vi "Gui_SetupExcitation_New.vi"(7 "Variant For Path":variant, 8 "error in (no error)":errorcluster, 11 "Variant":variant) -> (0 "error out":errorcluster caption="sortie d'erreur", 3 "Variant Output":variant)   [LabVIEW 2017]
uses:
  controls/SEQUENCE_Inputs.ctl
  controls/TRAPPING_Inputs.ctl
  controls/EXCIT_Inputs.ctl
  controls/DATA_Inputs.ctl
  controls/TIMING_Inputs.ctl
  controls/PROCESSING_Inputs.ctl
  controls/EXCIT_Form_Selector.ctl
  controls/EXPERT_Inputs.ctl
  controls/DIGIT_5122_Inputs.ctl
  <instrlib>/niScope/Controls/niScope trigger source.ctl
  controls/HSDIO_6541_Inputs.ctl
  <instrlib>/niHSDIO/niHSDIO.llb/niHSDIO_ctl Trigger Source Values (Ring).ctl
  controls/SOFTWARE_Inputs.ctl
  controls/AO_6711_Inputs.ctl
  controls/AWG_5421_Inputs.ctl
  <instrlib>/niFgen/niFgen.llb/niFgen_ctl Trigger Source Values (Ring).ctl
  controls/XML_Inputs.ctl
panel:
  in  "Excit Form":T1=enum."Swift"
  in  "CHECK":bool
  in  "TEST Text":string="script  excit1wfm\n    wait until scriptTrigger0\n    generate E1TwoSwift0p5f1000p0to1002p0a100and1003p0to1004p0a100d1200fs10\n    generate E2Chirp3p5f250p0to1000p0a50d800fs10\n    generate E3TwoSwift0p5f250p0to600p0a70and700p0to1000p0a50d1200fs10\n    generate E4Chirp3p5f250p0to1000p0a50d800fs10\n    generate E5Chirp3p5f250p0to1000p0a50d800fs40\nend script\n"
  in  "Waveforms Table":i32(listbox)
  out "Sampling Frequency":dbl=20.0
  out "Number of Ejects":u16=1
  out "Number of Excits":u16=3
  out "Script Text":string
  in  "SEQUENCE Inputs":T2={"TRAPPING Inputs"={"Number of Channels"=4, "Init Values"=[2.0, 5.0, 5.0, 2.0], "Opening Values"=[0.0, 0.0, 0.0, 0.0], "Trapping Values"=[2.0, 5.0, 5.0, 2.0], "Emptying Values"=[-5.0, -5.0, -5.0, -5.0], "Adiabatic ON"=FALSE, "Adiabatic Duration"=0, "Adiabatic Waveforms"=["Adiabatic_None_2_2_2000.bin", "Adiabatic_Ramp_5_0_2000.bin", "Adiabatic_DoubleRamp_5_0_2000.bin", "Adiabatic_RC_2_0_2000.bin"]}, "EXCIT Inputs"={"Number of Excitations"=1, "Script Text"="", "Table of Waveforms"=[]}, "DATA Inputs"={"Record Length"=8192, "Sample Rate"=4.0, "Data Type"=0, "Vertical Range"=0.0, "Acquisition Duration"=100000.0}, "TIMING Inputs"={"Number of Acquisitions "=1, "Number of Accumulations"=1, "Table of Waveforms"=[], "Script Text"=""}, "PROCESSING Inputs"={"Reference Mass"=300.0939, "Cyclotron Freq"=255.727, "Magnetron Freq"=0.001}} {"PROCESSING Inputs"."Magnetron Freq" format="%.5g"; "PROCESSING Inputs"."Cyclotron Freq" format="%.5g"; "PROCESSING Inputs"."Reference Mass" format="%.5g"; "TIMING Inputs"."Number of Accumulations" min=0 max=50 step=1; "TIMING Inputs"."Number of Acquisitions" min=1 max=10 step=1; "DATA Inputs"."Vertical Range" items=["0.2"=0.2, "0.4"=0.4, "1"=1.0, "2"=2.0, "4"=4.0, "10"=10.0]; "DATA Inputs"."Data Type" items=["I16", "DBL"]; "DATA Inputs"."Sample Rate" items=["1 MHz"=1000000.0, "2 MHz"=2000000.0, "5 MHz"=5000000.0, "10 MHz"=10000000.0, "20 MHz"=20000000.0, "25 MHz"=25000000.0, "50 MHz"=50000000.0, "100 MHz"=100000000.0]; "EXCIT Inputs"."Number of Excitations" min=1 max=10; "TRAPPING Inputs"."Trapping Values" min=-10.0 max=10.0; "TRAPPING Inputs"."Init Values" min=-10.0 max=10.0; "TRAPPING Inputs"."Emptying Values" min=-10.0 max=10.0; "TRAPPING Inputs"."Opening Values" min=-10.0 max=10.0}
  out "Script File":string
  in  "OK":bool
  # "GO_out"
  # "Gout"
  # "GI_in"
  # "Gin"
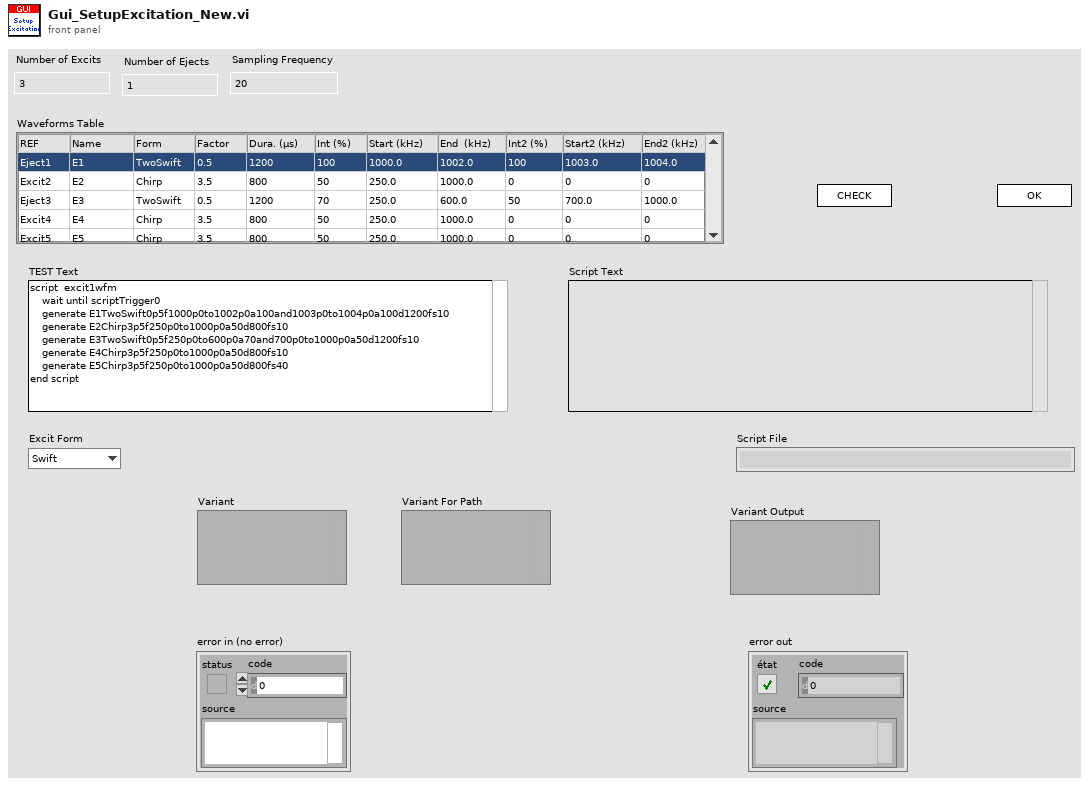
[diagram p1: front panel]
types:
  T1 = typedef "EXCIT_Form_Selector.ctl" = enum16{"Sinus", "Chirp", "Swift", "TwoSwift", "Ramp"}
  T2 = typedef "SEQUENCE_Inputs.ctl" = cluster{"TRAPPING Inputs":T3, "EXCIT Inputs":T4, "DATA Inputs":T5, "TIMING Inputs":T6, "PROCESSING Inputs":T7}
  T3 = typedef "TRAPPING_Inputs.ctl" = cluster{"Number of Channels":i32, "Init Values":dbl[], "Opening Values":dbl[], "Trapping Values":dbl[], "Emptying Values":dbl[], "Adiabatic ON":bool, "Adiabatic Duration":i32, "Adiabatic Waveforms":string[]}
  T4 = typedef "EXCIT_Inputs.ctl" = cluster{"Number of Excitations":i32, "Script Text":string, "Table of Waveforms":string[]}
  T5 = typedef "DATA_Inputs.ctl" = cluster{"Record Length":i32, "Sample Rate":dbl, "Data Type":u8, "Vertical Range":dbl, "Acquisition Duration":dbl}
  T6 = typedef "TIMING_Inputs.ctl" = cluster{"Number of Acquisitions ":i16, "Number of Accumulations":i16, "Table of Waveforms":string[], "Script Text":string}
  T7 = typedef "PROCESSING_Inputs.ctl" = cluster{"Reference Mass":dbl, "Cyclotron Freq":dbl, "Magnetron Freq":dbl}
  T8 = typedef "EXPERT_Inputs.ctl" = cluster{"DIGIT 5122 Inputs":T9, "HSDIO 6541 Inputs":T11, "SOFTWARE Inputs":T13, "AO 6711 Inputs":T14, "AWG 5421 Inputs":T15, "XML Inputs":T17}
  T9 = typedef "DIGIT_5122_Inputs.ctl" = cluster{"Sample Rate":dbl, "Resource Name":refnum<k15>, "Channel Name":string, "Trigger Source":T10, "Vertical Range":dbl, "Trigger Level":dbl}
  T10 = typedef "niScope trigger source.ctl" = string
  T11 = typedef "HSDIO_6541_Inputs.ctl" = cluster{"Resource Name":refnum<k15>, "Clock Rate":dbl, "Trigger Source":T12}
  T12 = typedef "niHSDIO_ctl Trigger Source Values (Ring).ctl" = string
  T13 = typedef "SOFTWARE_Inputs.ctl" = cluster{"Application Directory":path, "Software Version":string, "Data Path":path, "XML Path":path, "XML File Filter":string, "XML Saved Path":path, "Excit Scripts Path":path, "Excit Scripts File Filter":string, "Excit Waveforms Path":path, "Excit Waveforms File Filter":string, "Timing Scripts Path":path, "Timing Scripts File Filter":string, "Timing Waveforms Path":path, "Timing Waveforms File Filter":string, "Trapping Waveforms Path":path, "Trapping Waveforms File Filter":string}
  T14 = typedef "AO_6711_Inputs.ctl" = cluster{"Physical Channels":tag, "Min Voltage":dbl, "Max Voltage":dbl, "Trigger Source":tag, "Counter":tag}
  T15 = typedef "AWG_5421_Inputs.ctl" = cluster{"Resource Name":refnum<k15>, "Sample Rate":dbl, "Trigger Type":u16, "Trigger Source":T16, "Waveform Gain":dbl, "Digital Filter ON":bool}
  T16 = typedef "niFgen_ctl Trigger Source Values (Ring).ctl" = string
  T17 = typedef "XML_Inputs.ctl" = cluster{"Version Tag Name":string, "Version String":string}
  T18 = typedef "EXCIT_Table.ctl" = cluster{"Number of Excits":u16, "Number of Ejects":u16, "Sampling Frequency":dbl, "Waveforms Table":string[][]}
  T19 = typedef "LVPoint32TypeDef.ctl" = cluster{"Horizontal":i32, "Vertical":i32}
  T20 = typedef "LVRowAndColumnTypeDef.ctl" = cluster{"Row":i32, "Column":i32}
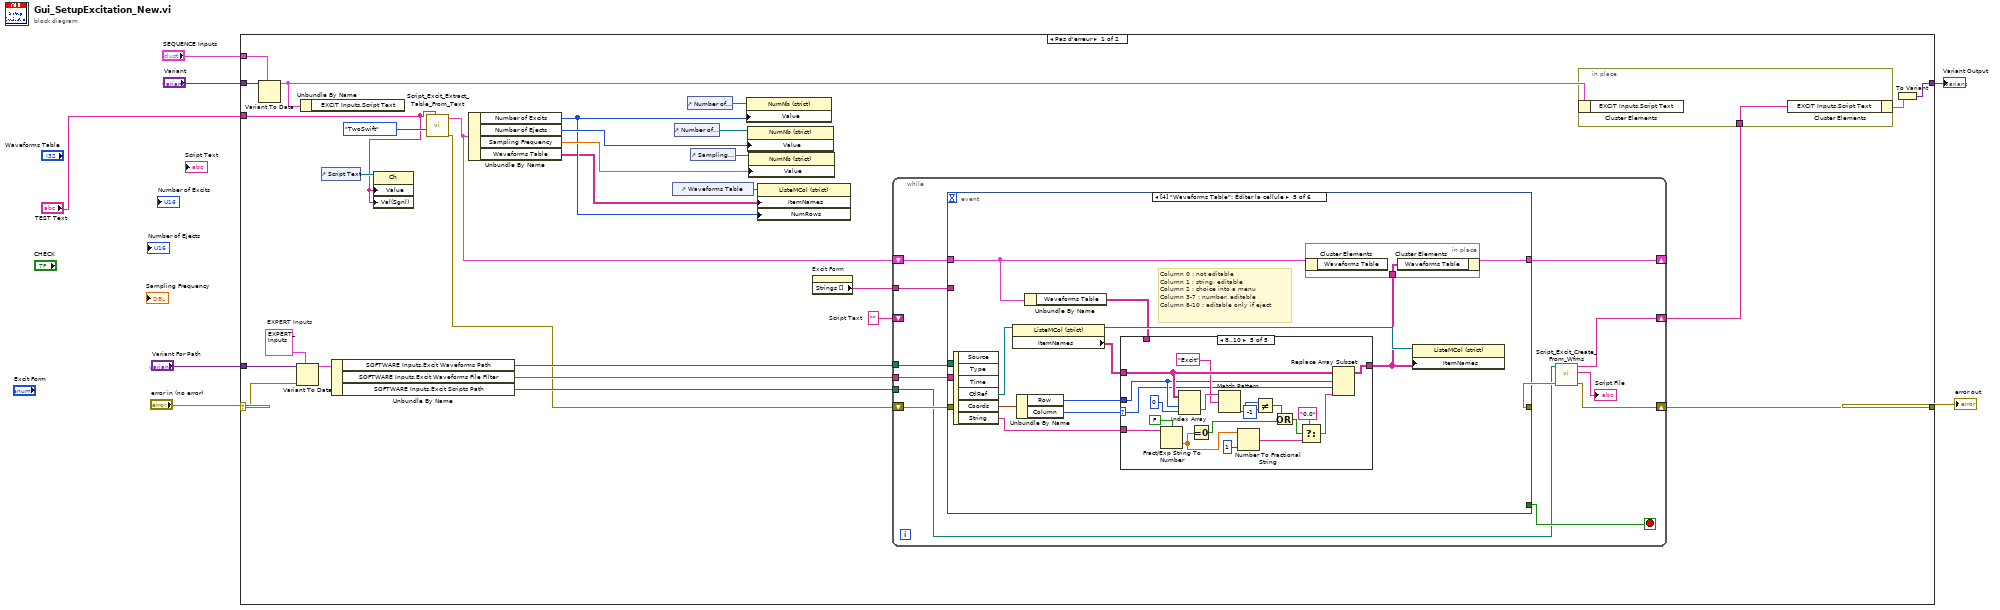
[diagram p0: block diagram]
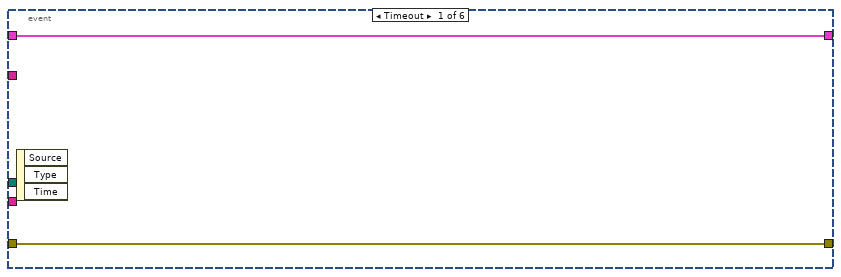
[diagram p2: hidden frame]
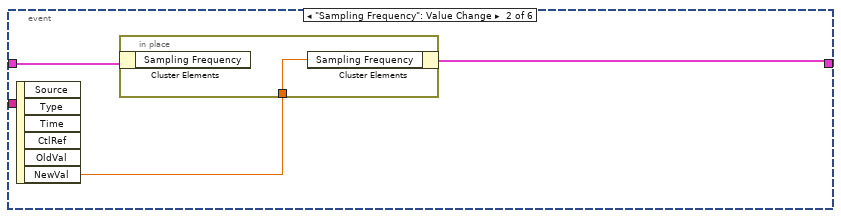
[diagram p3: hidden frame]
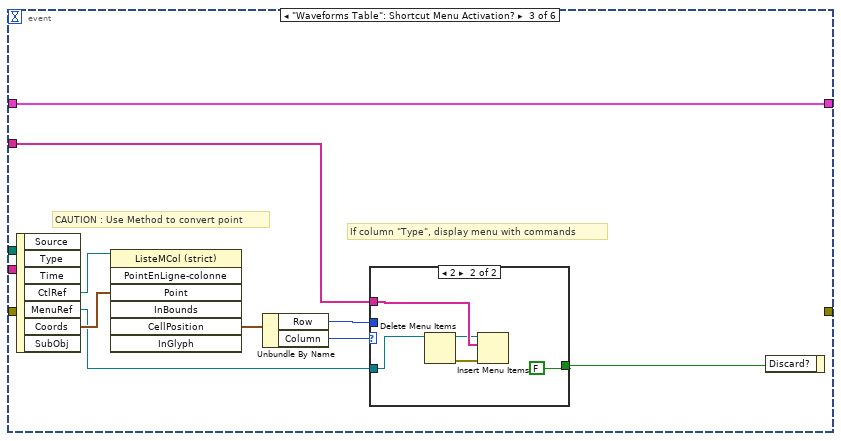
[diagram p4: hidden frame]
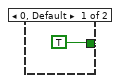
[diagram p5: hidden frame]
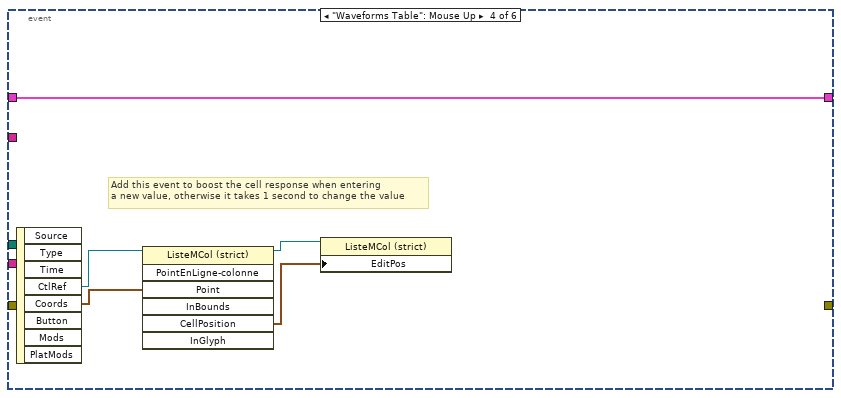
[diagram p6: hidden frame]
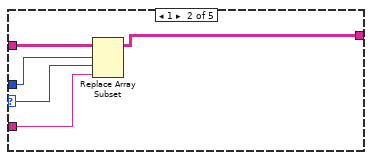
[diagram p8: hidden frame]
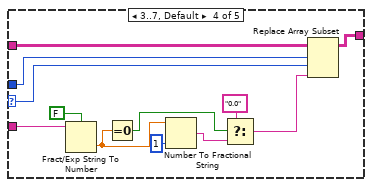
[diagram p10: hidden frame]
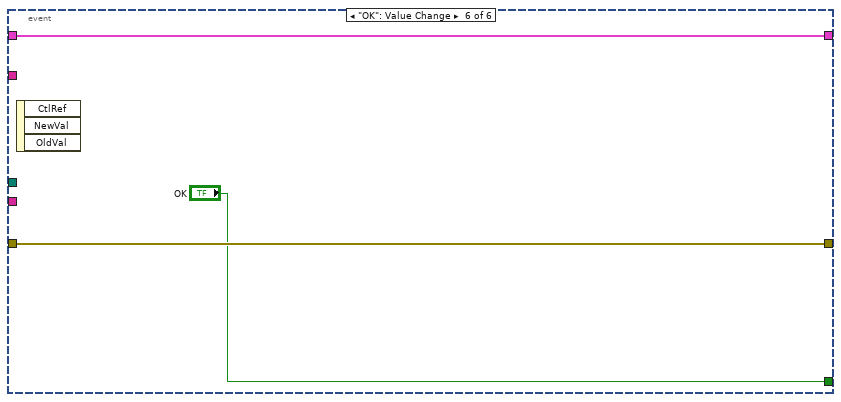
[diagram p11: hidden frame]
diagram:
  n1 = case shown="Pas d'erreur" "error in (no error)" {
    selector: "error in (no error)" -> [w20 w130]
    tunnel: [w36 w130] -> w6
    tunnel: "Variant" -> [w30 w129]
    tunnel: "Variant For Path" -> [w33 _]
    tunnel: [w27 w129] -> w3
    tunnel: "SEQUENCE Inputs" -> [w25 _]
    tunnel: "TEST Text" -> [w13 _]
    frame No Error {
      w11 = ""  # Script Text
      w35 = T8 {"DIGIT 5122 Inputs"={"Sample Rate"=1.0, "Resource Name"="Digitizer", "Channel Name"="0", "Trigger Source"="VAL_EXTERNAL", "Vertical Range"=10.0, "Trigger Level"=3.0}, "HSDIO 6541 Inputs"={"Resource Name"="SequencerHSDIO", "Clock Rate"=1000000.0, "Trigger Source"="PFI0"}, "SOFTWARE Inputs"={"Application Directory"=path "D:/S.O.F.T.S/LABVIEW/PIL", "Software Version"="1.0.0", "Data Path"=path "D:/PIRENEA/DATA", "XML Path"=path "D:/PIRENEA/DATA", "XML File Filter"="*.xml", "XML Saved Path"=path "D:/PIRENEA/DATA", "Excit Scripts Path"=path "D:/PIRENEA/EXCIT_SCRIPTS", "Excit Scripts File Filter"="*.txt", "Excit Waveforms Path"=path "D:/PIRENEA/EXCIT_WFMS", "Excit Waveforms File Filter"="*.bin", "Timing Scripts Path"=path "D:/PIRENEA/SEQUENCE_SCRIPTS", "Timing Scripts File Filter"="*.txt", "Timing Waveforms Path"=path "D:/PIRENEA/SEQUENCE_WFMS", "Timing Waveforms File Filter"="*.bin", "Trapping Waveforms Path"=path "D:/PIRENEA/TRAPPING_WFMS", "Trapping Waveforms File Filter"="*.bin"}, "AO 6711 Inputs"={"Physical Channels"="AnalogOutput/ao0:3", "Min Voltage"=-10.0, "Max Voltage"=10.0, "Trigger Source"="/AnalogOutput/PFI0", "Counter"="AnalogOutput/ctr0"}, "AWG 5421 Inputs"={"Resource Name"="WaveformGenerator", "Sample Rate"=0.0, "Trigger Type"=4, "Trigger Source"="PFI0", "Waveform Gain"=0.31, "Digital Filter ON"=TRUE}, "XML Inputs"={"Version Tag Name"="XML_Version", "Version String"="1.0"}}  # EXPERT Inputs
      n2 = Variant To Data(type=w25, Variant=w30) -> (data=w26:T2)  [unwired: 1 in, 1 out]
      n3 = Variant To Data(error in=w20, type=w35, Variant=w33) -> (data=w34:T8)  [unwired: 1 out]
      n4 = Unbundle By Name(w26) -> ()  [unwired: 1 out]
      n5 = control-ref of="Script Text"() -> (w22:refnum<vi>)
      n6 = Unbundle By Name(w34) -> ("SOFTWARE Inputs.Excit Waveforms Path"=w23:path, "SOFTWARE Inputs.Excit Waveforms File Filter"=w32:string, "SOFTWARE Inputs.Excit Scripts Path"=w31:path)
      n7 = property class="Ch"(reference=w22, "Value"=w13, "Val(Sgnl)"=w13) -> ()  [unwired: 1 in, 2 out]
      n8 = call "Script_Excit_Extract_Table_From_Text.vi"("Excit Text"=w13, "Excit Form"=EXCIT_Form_Selector."TwoSwift") -> ("error out"=w21:errorcluster, "EXCIT Table"=w9:T18)  [unwired: 6 in, 2 out]
      n9 = Unbundle By Name(w9) -> ("Number of Excits"=w12:u16, "Number of Ejects"=w17:u16, "Sampling Frequency"=w15:dbl, "Waveforms Table"=w10:string[][])
      n10 = control-ref of="Waveforms Table"() -> (w14:refnum<vi>)
      n11 = control-ref of="Number of Ejects"() -> (w18:refnum<vi>)
      n12 = control-ref of="Number of Excits"() -> (w19:refnum<vi>)
      n13 = control-ref of="Sampling Frequency"() -> (w16:refnum<vi>)
      n14 = property class="NumNb (strict)"(reference=w19, "Value"=w12) -> ()  [unwired: 1 in, 2 out]
      n15 = property class="NumNb (strict)"(reference=w18, "Value"=w17) -> ()  [unwired: 1 in, 2 out]
      n16 = property class="NumNb (strict)"(reference=w16, "Value"=w15) -> ()  [unwired: 1 in, 2 out]
      n17 = property class="ListeMCol (strict)"(reference=w14, "ItemNames"=w10, "NumRows"=w12) -> ()  [unwired: 1 in, 2 out]
      n18 = property on="Excit Form" class="Énum (strict)"() -> ("Strings []"=w8:string[])  [unwired: 2 in, 2 out]
      n19 = while {
        shift-right: [w43] -> w36
        shift-left: w21 -> [w48]
        shift-right: [w40] -> _
        shift-left: w9 -> [w47]
        tunnel: w23 -> [w46]
        tunnel: w32 -> [w45]
        tunnel: w31 -> [w38]
        shift-right: [w41] -> w29
        shift-left: w11 -> [_]
        tunnel: w8 -> [w37]
        stop <- w39 stop-if-true
        n20 = event shown="[4] \"Waveforms Table\": Éditer la cellule" {
          selector: _ -> [_ _ _ _ _ _]
          dyn-events: _ -> [_ _ _ _ _ _]
          timeout: _ -> [_ _ _ _ _ _]
          tunnel: w48 -> [w50 _ _ _ _ w127]
          tunnel: [w50 _ _ _ _ w127] -> w44
          tunnel: w47 -> [w49 w53 w55 w70 w79 w125]
          tunnel: [w49 w51 w55 w70 w75 w125] -> w40
          tunnel: w46 -> [_ _ _ _ _ _]
          tunnel: w45 -> [_ _ _ _ _ _]
          tunnel: [_ _ _ _ _ "OK"] -> w39
          tunnel: w37 -> [_ _ w61 _ _ _]
          event Timeout {
            n21 = event-data() -> ()  [unwired: 1 in, 3 out]
          }
          event "Sampling Frequency": Value Change {
            n22 = event-data() -> ("NewVal"=w52:dbl)  [unwired: 1 in, 5 out]
            n23 = in-place {
              in-place-border: w52 -> [w54]
              n24 = in-place-cluster #1(w53) -> ()  [unwired: 1 out]
              n25 = in-place-cluster #1("Sampling Frequency"=w54) -> (w51:T18)
            }
          }
          event "Waveforms Table": Shortcut Menu Activation? {
            # "If column \"Type\", display menu with commands"
            # "CAUTION : Use Method to convert point"
            n26 = event-data() -> ("CtlRef"=w58:refnum<vi>, "MenuRef"=w57:refnum<k9>, "Coords"=w60:T19)  [unwired: 1 in, 4 out]
            n27 = invoke on="Nœud de méthode" class="ListeMCol (strict)" method="PointEnLigne-colonne"(reference=w58, "Point"=w60) -> ("CellPosition"=w59:T20)  [unwired: 5 in, 6 out]
            n28 = Unbundle By Name(w59) -> ("Row"=w62:i32, "Column"=w63:i32)
            n29 = case shown="2" w63 {
              tunnel: [TRUE FALSE] -> w56
              tunnel: w62 -> [_ _]
              tunnel: w61 -> [_ w68]
              tunnel: w57 -> [_ w65]
              frame 0, Default {
              }
              frame 2 {
                n30 = Delete Menu Items(9:w65) -> (0:w67:errorcluster, 3:w66:refnum<k9>)  [unwired: 3 in]
                n31 = Insert Menu Items(6:w67, 8:w68, 9:w66) -> ()  [unwired: 3 in, 3 out]
              }
            }
            n32 = event-data("Discard?"=w56) -> ()  [unwired: 1 in, 1 out]
          }
          event "Waveforms Table": Mouse Up {
            # "Add this event to boost the cell response when entering\na new value, otherwise it takes 1 second to change the value"
            n33 = event-data() -> ("CtlRef"=w71:refnum<vi>, "Coords"=w72:T19)  [unwired: 1 in, 6 out]
            n34 = invoke class="ListeMCol (strict)" method="PointEnLigne-colonne"(reference=w71, "Point"=w72) -> (reference out=w74:refnum<vi>, "CellPosition"=w73:T20)  [unwired: 5 in, 5 out]
            n35 = property class="ListeMCol (strict)"(reference=w74, "EditPos"=w73) -> ()  [unwired: 1 in, 2 out]
          }
          event "Waveforms Table": Edit Cell {
            # "Column 0 : not editable\nColumn 1 : string, editable\nColumn 2 : choice into a menu\nColumn 3-7 : number, editable\nColumn 8-10 : editable only if eject"
            n36 = event-data() -> ("CtlRef"=w76:refnum<vi>, "Coords"=w78:T20, "String"=w77:string)  [unwired: 1 in, 3 out]
            n37 = property class="ListeMCol (strict)"(reference=w76) -> (reference out=w82:refnum<vi>, "ItemNames"=w85:string[][])  [unwired: 1 in, 1 out]
            n38 = Unbundle By Name(w78) -> ("Row"=w84:i32, "Column"=w83:i32)
            n39 = Unbundle By Name(w79) -> ("Waveforms Table"=w81:string[][])
            n40 = case shown="8..10" w83 {
              selector: w83 -> [_ w88 _ w94 w106]
              tunnel: w77 -> [_ w92 _ w105 w124]
              tunnel: w85 -> [_ w90 _ w96 w116]
              tunnel: w84 -> [_ w89 _ w95 w107]
              tunnel: [w87 w91 w93 w104 w123] -> w80
              tunnel: w81 -> [w87 _ w93 _ _]
              frame 0 {
              }
              frame 1 {
                n41 = Replace Array Subset(array=w90, new element=w92, index (row)=w89, index (col)=w88) -> (w91:string[][])
              }
              frame 2 {
              }
              frame 3..7, Default {
                n42 = Fract/Exp String To Number(use system decimal point (T)=FALSE ("utiliser le séparateur décimal du système (V)"), string=w105) -> (number=w100:dbl)  [unwired: 2 in, 1 out]
                n43 = Equal To 0?(x=w100) -> (x = 0?=w97:bool)
                n44 = Number To Fractional String(number=w100, precision (6)=i16 1 ("précision (6)")) -> (F-format string=w98:string)  [unwired: 2 in]
                n45 = Select(t="0.0", s=w97, f=w98) -> (s? t:f=w102:string)
                n46 = Replace Array Subset(array=w96, new element=w102, index (row)=w95, index (col)=w94) -> (w104:string[][])
              }
              frame 8..10 {
                n47 = Fract/Exp String To Number(use system decimal point (T)=FALSE ("utiliser le séparateur décimal du système (V)"), string=w124) -> (number=w119:dbl)  [unwired: 2 in, 1 out]
                n48 = Index Array(array=w116, index (row)=w107, index (col)=0 ("indice désactivé (col)")) -> (element=w114:string)
                n49 = Equal To 0?(x=w119) -> (x = 0?=w111:bool)
                n50 = Match Pattern(string=w114, regular expression="Excit" ("expression régulière")) -> (offset past match=w110:i32)  [unwired: 1 in, 3 out]
                n51 = Number To Fractional String(number=w119, precision (6)=i16 1 ("précision (6)")) -> (F-format string=w117:string)  [unwired: 2 in]
                n52 = Not Equal?(x=w110, y=-1) -> (x != y?=w108:bool)
                n53 = Or(x=w108, y=w111) -> (x .or. y?=w112:bool)
                n54 = Select(t="0.0", s=w112, f=w117) -> (s? t:f=w121:string)
                n55 = Replace Array Subset(array=w116, new element=w121, index (row)=w107, index (col)=w106) -> (w123:string[][])
              }
            }
            n56 = in-place {
              in-place-border: w80 -> [w86]
              n57 = in-place-cluster #2(w79) -> ()  [unwired: 1 out]
              n58 = in-place-cluster #2("Waveforms Table"=w86) -> (w75:T18)
            }
            n59 = property class="ListeMCol (strict)"(reference=w82, "ItemNames"=w80) -> ()  [unwired: 1 in, 2 out]
          }
          event "OK": Value Change {
            n60 = event-data() -> ()  [unwired: 1 in, 3 out]
          }
        }
        n61 = call "Script_Excit_Create_From_Wfms.vi"("error in (no error)"=w44, "Script Path"=w38) -> ("error out"=w43:errorcluster, "Script File"=→"Script File":string, "Script Text"=w41:string)  [unwired: 7 in]
      }
      n62 = in-place {
        in-place-border: w29 -> [w128]
        n63 = in-place-cluster #3(w26) -> ()  [unwired: 1 out]
        n64 = in-place-cluster #3("EXCIT Inputs.Script Text"=w128) -> (w28:T2)
      }
      n65 = To Variant(anything=w28) -> (Variant=w27:variant)
    }
    frame Error {
    }
  }
  "error out" <- w6
  "Variant Output" <- w3
